vi "FTW-JSON-Construct-FromPointer.vi"(5 "JSON Object Pointer":i64, 11 "error in":errorcluster) -> (4 "JSON Object":refnum<class "FTW-JSON.lvclass">, 15 "error out":errorcluster)   [LabVIEW 2013, in "FTW-JSON.lvclass"]
uses:
  FTW-JSON.lvclass
  FTW-JSON.lvclass/FTW-JSON.ctl
panel:
  # "Inputs"
  # "Outputs"
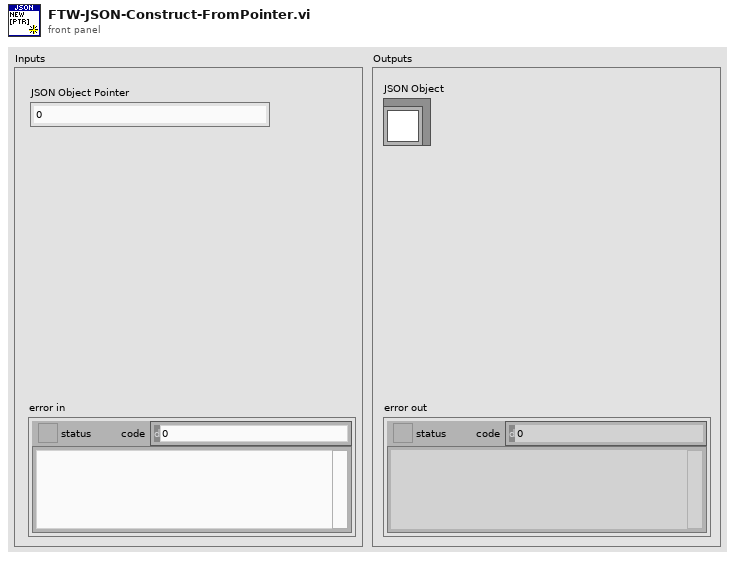
[diagram p1: front panel]
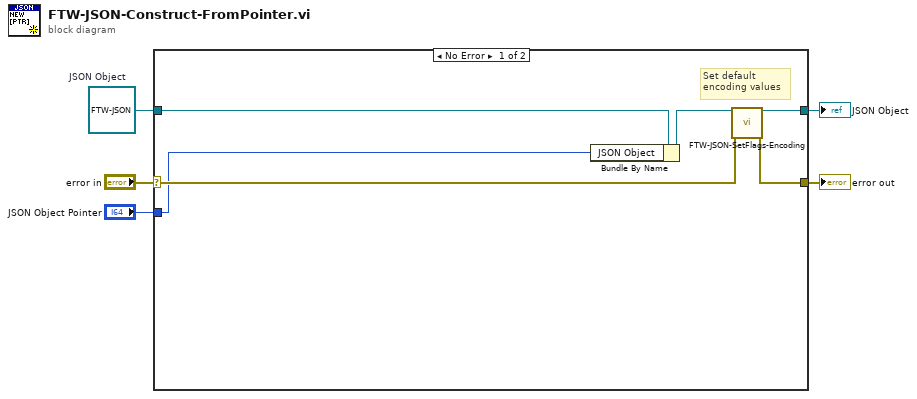
[diagram p0: block diagram]
diagram:
  w4 = refnum<class "FTW-JSON.lvclass"> refnum  # JSON Object
  n1 = case shown="No Error" "error in" {
    selector: "error in" -> [w10 w13]
    tunnel: [w6 w13] -> w5
    tunnel: [w7 w12] -> w3
    tunnel: w4 -> [w11 w12]
    tunnel: "JSON Object Pointer" -> [w9 _]
    frame No Error {
      # "Set default\nencoding values"
      n2 = Bundle By Name(cluster=w11, "JSON Object"=w9) -> (w8:refnum<class "FTW-JSON.lvclass">)
      n3 = call "FTW-JSON-SetFlags-Encoding.vi"("JSON Object"=w8, "error in"=w10) -> ("JSON Object out"=w7:refnum<class "FTW-JSON.lvclass">, "error out"=w6:errorcluster)  [unwired: 12 in]
    }
    frame Error {
    }
  }
  "error out" <- w5
  "JSON Object" <- w3
